vi "Save Changes (Hardware).vi"(6 "Remote Timeout (300,000 ms)":u32=300000, 8 "error in (no error)":errorcluster, 11 "Resource in":refnum<k20>) -> (0 "error out":errorcluster, 1 "Changes Require Restart":bool, 2 "Detailed Result":string, 3 "Resource out":refnum<k20>)   [LabVIEW 2014, in "nisyscfg.lvlib"]
doc: "Writes and saves property changes on a device. Save Changes (Hardware) VI wires into the Hardware Property node where property changes are selected."
uses:
  nisyscfg.lvlib
  Error Cluster From Error Code.vi
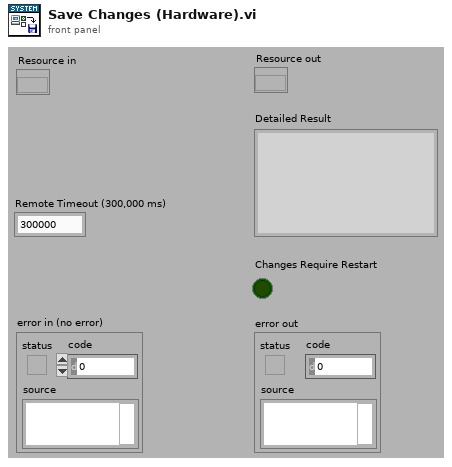
[diagram p1: front panel]
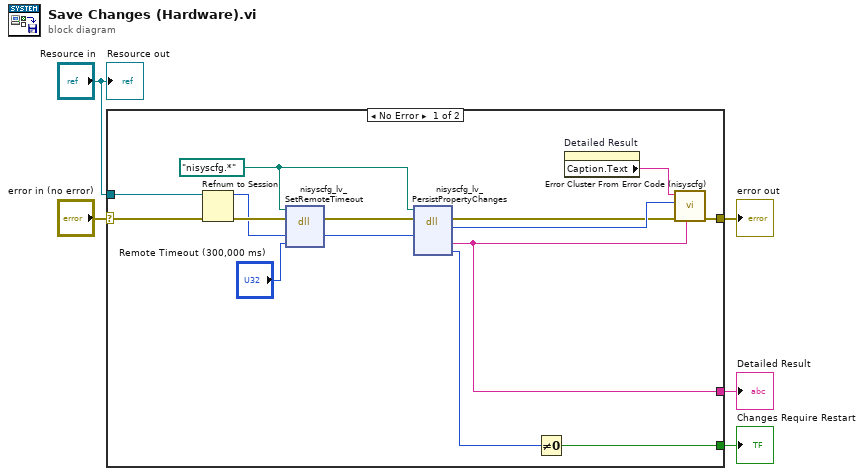
[diagram p0: block diagram]
diagram:
  n1 = case shown="No Error" "error in (no error)" {
    selector: "error in (no error)" -> [w12 w21]
    tunnel: [w18 w21] -> w5
    tunnel: [w6 _] -> w3
    tunnel: "Resource in" -> [w11 _]
    tunnel: [w8 _] -> w1
    frame No Error {
      w10 = path "nisyscfg.*" ("path in")
      n2 = Refnum to Session(4:w12, 7:w11) -> (0:w17:errorcluster, 3:w15:u64)
      n3 = dll-call lib="nisyscfg.*" fn="nisyscfg_lv_SetRemoteTimeout" label="SetRemoteTimeout"(path in=w10, error in=w17, "item"=w15, "connectTimeout"="Remote Timeout (300,000 ms)") -> (error out=w16:errorcluster, "item"=w13:u64)  [unwired: 1 in, 3 out]
      n4 = dll-call lib="nisyscfg.*" fn="nisyscfg_lv_PersistPropertyChanges" label="nisysPersistPropertyChangesLV"(path in=w10, error in=w16, "item"=w13) -> (error out=w19:errorcluster, "status"=w20:i32, "detailed result"=w6:string, "requiresRestart"=w9:u8)  [unwired: 1 in, 4 out]
      n5 = Not Equal To 0?(x=w9) -> (x != 0?=w8:bool)
      n6 = property on="Detailed Result" class="Str"() -> ("Caption.Text"=w7:string)  [unwired: 2 in, 2 out]
      n7 = call "Error Cluster From Error Code (nisyscfg).vi"("Details String"=w6, "error in (no error)"=w19, "Error Code (0)"=w20, "Details Caption"=w7) -> ("error out"=w18:errorcluster)  [unwired: 7 in]
    }
    frame Error {
    }
  }
  "error out" <- w5
  "Detailed Result" <- w3
  "Changes Require Restart" <- w1
  "Resource out" <- "Resource in"
